vi "Open API Reference.vi"(8 "error in (no error)":errorcluster) -> (0 "error out":errorcluster, 3 "Execution API Out":refnum<class "Execution API.lvclass">)   [LabVIEW 2020, in "Execution API.lvclass"]
doc: "Initializes the API and obtains a reference. The reference should be closed using the Close API Reference.vi when it is no longer needed."
uses:
  Execution API.lvclass
  Core/Result/Result.ctl
  Core/Result/Status.ctl
  Core/Result/Type.ctl
  Plugin/Plugin.lvclass
  Execution API.lvclass/Execution API.ctl
  Single Thread Test Runner/Single Thread Test Runner.lvclass
  C:/git/astemes-lunit/source/Framework/Test Runner/Test Runner.lvclass
  Core/Result/Result.lvlib
  C:/git/astemes-lunit/source/Framework/Single Thread Test Runner/Single Thread Test Runner.lvclass
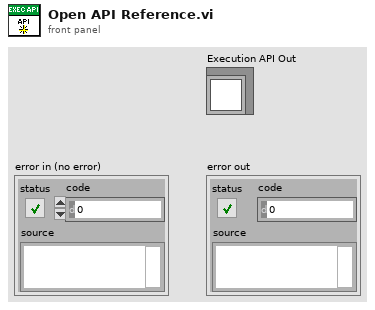
[diagram p1: front panel]
types:
  T1 = typedef "Result.lvlib/Result.ctl" = cluster{"Name":string, "Description":string, "Status":T2, "Result Type":T3, "Execution Time":dbl, "Data":cluster{"Expected":variant, "Actual":variant, "Delta":variant}}
  T2 = typedef "Result.lvlib/Status.ctl" = enum16{"", "Passed", "Failed", "Error", "Skipped", "Setup Error", "Broken", "Teardown Error"}
  T3 = typedef "Result.lvlib/Type.ctl" = enum16{"Test Case", "Test Suite", "Test Run", "Pass", "Fail", "Skip", "Pass if", "Fail if", "Pass if Error", "Fail if Error", "Pass if Equal", "Fail if Equal"}
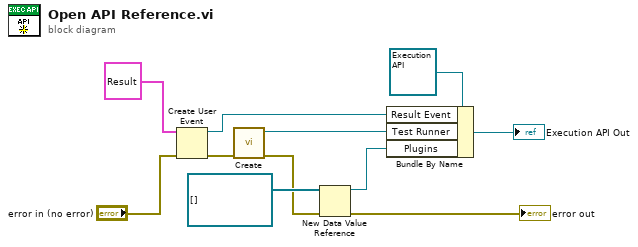
[diagram p0: block diagram]
diagram:
  n1 = Create User Event(user event datatype=T1 {"Name"="", "Description"="", "Status"=enum."Passed", "Result Type"=enum."Test Suite", "Execution Time"=0.0, "Data"={"Expected"=variant, "Actual"=variant, "Delta"=variant}} ("Result"), error in="error in (no error)") -> (user event=w3:refnum<user-event>, error out=w10:errorcluster)
  n2 = call "Create.vi"("error in (no error)"=w10) -> ("error out"=w5:errorcluster, "Single Thread Test Runner out"=w11:refnum<class "Single Thread Test Runner.lvclass">)  [unwired: 9 in]
  n3 = New Data Value Reference(data value=refnum<class "Plugin.lvclass">[] [] ("Plugins"), error in=w5) -> (data value reference=w6:refnum<data-value>, error out=→"error out":errorcluster)
  n4 = Bundle By Name(cluster=refnum<class "Execution API.lvclass"> refnum ("LUnit API.lvclass"), "Result Event"=w3, "Test Runner"=w11, "Plugins"=w6) -> (→"Execution API Out":refnum<class "Execution API.lvclass">)
